vi "Conf Alarm.vi"(0 "VISA Resource Name":refnum<visa-resource-name>, 1 "Enable Alarm? (T:Enable)":bool=TRUE, 2 "Set/Check (F:Set)":bool, 3 "Polarity (T:Positive)":bool=TRUE, 4 "Mode (F:Track)":bool, 5 "error in (no error)":errorcluster, 6 "Alarm(s) (2:Both)":enum16{"Lower", "Upper", "Both"}(ring)=enum."Both", 7 "Lower Limit (0)":dbl format="%.2f", 8 "Channel List(empty)":string, 9 "Upper Limit (0)":dbl format="%.2f", 10 "Check (2:Lower Limit)":T1(ring)=enum."Lower Limit", 11 "Clear Bit (5:None)":enum16{"1", "2", "3", "4", "All", "None"}(ring)=enum."None", 13 "Output # (1)":enum16{"1", "2", "3", "4"}(ring)) -> (14 "VISA Resource Name Out":refnum<visa-resource-name>, 16 "Configuration?":string, 19 "error out":errorcluster)   [LabVIEW 2012, in "Agilent 34970.lvlib"]
doc: "This VI lets you configure or check alarms on the specified analog channels."
uses:
  <instrlib>/Agilent 34970/Agilent 34970.lvlib
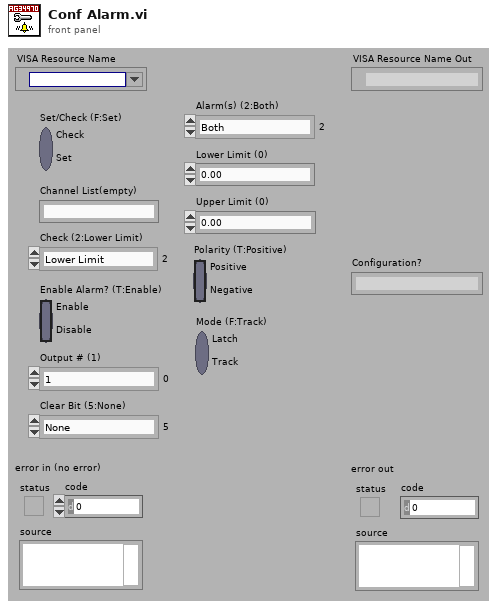
[diagram p1: front panel]
types:
  T1 = enum16{"Lower State", "Upper State", "Lower Limit", "Upper Limit", "Alarm #", "Polarity", "Mode"}
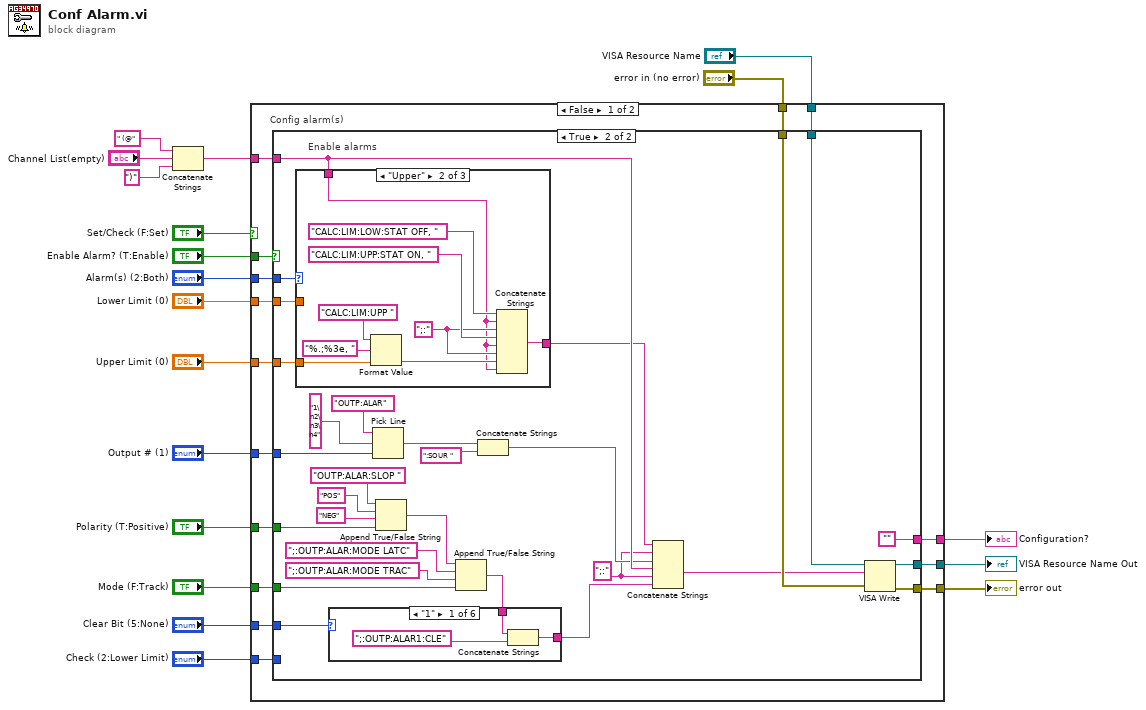
[diagram p0: block diagram]
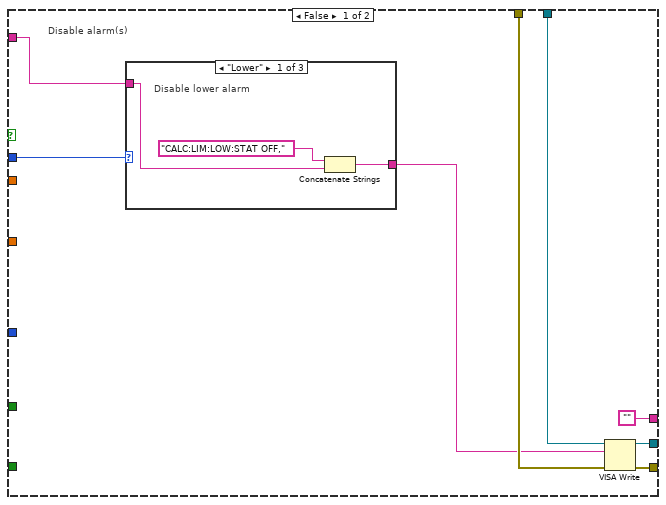
[diagram p2: hidden frame]
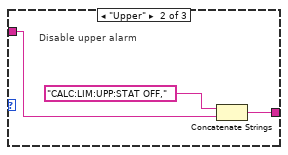
[diagram p3: hidden frame]
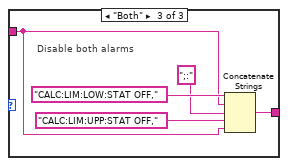
[diagram p4: hidden frame]
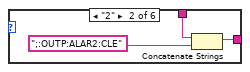
[diagram p5: hidden frame]
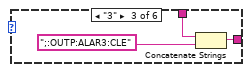
[diagram p6: hidden frame]
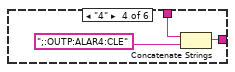
[diagram p7: hidden frame]
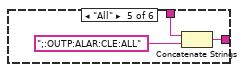
[diagram p8: hidden frame]
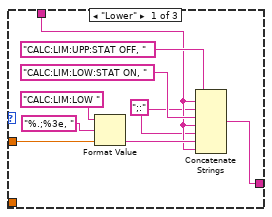
[diagram p10: hidden frame]
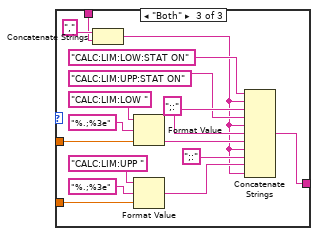
[diagram p11: hidden frame]
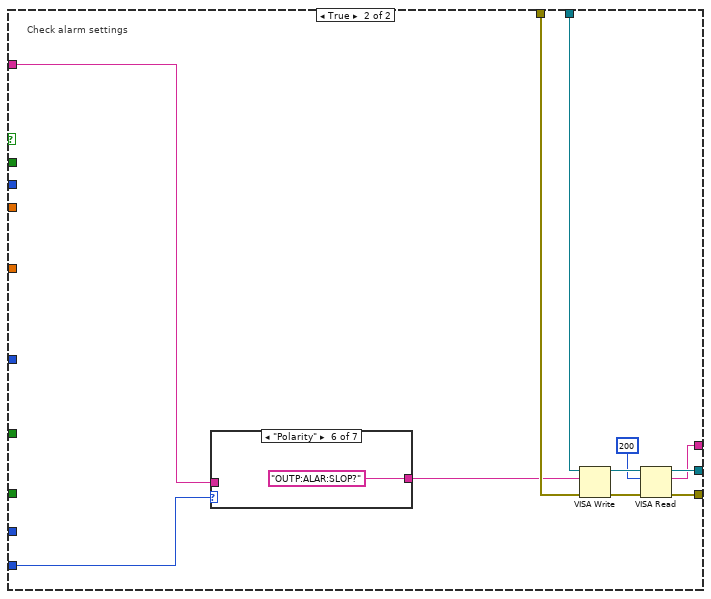
[diagram p12: hidden frame]
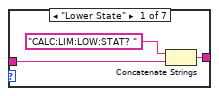
[diagram p13: hidden frame]
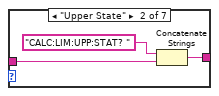
[diagram p14: hidden frame]
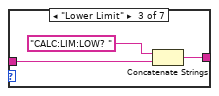
[diagram p15: hidden frame]
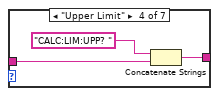
[diagram p16: hidden frame]
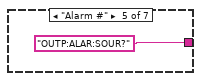
[diagram p17: hidden frame]
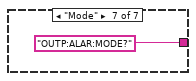
[diagram p18: hidden frame]
diagram:
  n1 = Concatenate Strings(" (@", "Channel List(empty)", ")") -> (w16:string)
  n2 = case shown="False" "Set/Check (F:Set)" {
    tunnel: w16 -> [w34 w135]
    tunnel: "error in (no error)" -> [w33 w140]
    tunnel: "VISA Resource Name" -> [w32 w139]
    tunnel: [w31 w138] -> w4
    tunnel: [w30 w136] -> w3
    tunnel: [w29 w137] -> w15
    tunnel: "Alarm(s) (2:Both)" -> [w28 _]
    tunnel: "Lower Limit (0)" -> [w27 _]
    tunnel: "Upper Limit (0)" -> [w26 _]
    tunnel: "Output # (1)" -> [w25 _]
    tunnel: "Polarity (T:Positive)" -> [w24 _]
    tunnel: "Mode (F:Track)" -> [w23 _]
    tunnel: "Clear Bit (5:None)" -> [w22 _]
    tunnel: "Check (2:Lower Limit)" -> [w21 w133]
    tunnel: "Enable Alarm? (T:Enable)" -> [w20 _]
    frame False {
      # "Config alarm(s)"
      n3 = case shown="True" w20 {
        tunnel: w34 -> [w37 w62]
        tunnel: w33 -> [w39 w82]
        tunnel: w32 -> [w38 w81]
        tunnel: [w41 w80] -> w31
        tunnel: [w40 w79] -> w30
        tunnel: ["" ""] -> w29
        tunnel: w28 -> [w36 w77]
        tunnel: w27 -> [_ w76]
        tunnel: w26 -> [_ w75]
        tunnel: w25 -> [_ w72]
        tunnel: w24 -> [_ w68]
        tunnel: w23 -> [_ w66]
        tunnel: w22 -> [_ w65]
        tunnel: w21 -> [_ _]
        frame False {
          # "Disable alarm(s)"
          n4 = case shown="\"Lower\"" w36 {
            tunnel: [w44 w47 w50] -> w35
            tunnel: w37 -> [w43 w46 w49]
            frame "Lower" {
              # "Disable lower alarm"
              n5 = Concatenate Strings("CALC:LIM:LOW:STAT OFF,", w43) -> (w44:string)
            }
            frame "Upper" {
              # "Disable upper alarm"
              n6 = Concatenate Strings("CALC:LIM:UPP:STAT OFF,", w46) -> (w47:string)
            }
            frame "Both" {
              # "Disable both alarms"
              n7 = Concatenate Strings("CALC:LIM:LOW:STAT OFF,", w49, ";:", "CALC:LIM:UPP:STAT OFF,", w49) -> (w50:string)
            }
          }
          n8 = VISA Write(VISA resource name=w38, write buffer=w35, error in (no error)=w39) -> (VISA resource name out=w41:refnum<visa-resource-name>, error out=w40:errorcluster)  [unwired: 1 out]
        }
        frame True {
          w60 = ";:"
          # "Enable alarms"
          n9 = case shown="\"Upper\"" w77 {
            tunnel: w76 -> [w106 _ w130]
            tunnel: w75 -> [_ w112 w129]
            tunnel: w62 -> [w101 w108 w119]
            tunnel: [w103 w111 w117] -> w59
            frame "Lower" {
              w100 = ";:"
              n10 = Format Value(string ("")="CALC:LIM:LOW ", format string="%.;%3e, ", value (0)=w106) -> (output string=w105:string)
              n11 = Concatenate Strings("CALC:LIM:UPP:STAT OFF, ", w101, w100, "CALC:LIM:LOW:STAT ON, ", w101, w100, w105, w101) -> (w103:string)
            }
            frame "Upper" {
              w109 = ";:"
              n12 = Format Value(string ("")="CALC:LIM:UPP ", format string="%.;%3e, ", value (0)=w112) -> (output string=w114:string)
              n13 = Concatenate Strings("CALC:LIM:LOW:STAT OFF, ", w108, w109, "CALC:LIM:UPP:STAT ON, ", w108, w109, w114, w108) -> (w111:string)
            }
            frame "Both" {
              w123 = ";:"
              n14 = Concatenate Strings(",", w119) -> (w118:string)
              n15 = Format Value(string ("")="CALC:LIM:LOW ", format string="%.;%3e", value (0)=w130) -> (output string=w126:string)
              n16 = Format Value(string ("")="CALC:LIM:UPP ", format string="%.;%3e", value (0)=w129) -> (output string=w124:string)
              n17 = Concatenate Strings("CALC:LIM:LOW:STAT ON", w118, w123, "CALC:LIM:UPP:STAT ON", w118, w123, w126, w118, ";:", w124, w118) -> (w117:string)
            }
          }
          n18 = Pick Line(string ("")="OUTP:ALAR", multi-line string="1\n2\n3\n4", line index=w72) -> (output string=w71:string)
          n19 = Append True/False String(1:w68, 2:"NEG", 3:"POS", 4:"OUTP:ALAR:SLOP ") -> (0:w67:string)
          n20 = Append True/False String(1:w66, 2:";:OUTP:ALAR:MODE TRAC", 3:";:OUTP:ALAR:MODE LATC", 4:w67) -> (0:w64:string)
          n21 = case shown="\"1\"" w65 {
            tunnel: w64 -> [w85 w87 w90 w93 w96 w98]
            tunnel: [w83 w86 w89 w92 w95 w98] -> w63
            frame "1" {
              n22 = Concatenate Strings(w85, ";:OUTP:ALAR1:CLE") -> (w83:string)
            }
            frame "2" {
              n23 = Concatenate Strings(w87, ";:OUTP:ALAR2:CLE") -> (w86:string)
            }
            frame "3" {
              n24 = Concatenate Strings(w90, ";:OUTP:ALAR3:CLE") -> (w89:string)
            }
            frame "4" {
              n25 = Concatenate Strings(w93, ";:OUTP:ALAR4:CLE") -> (w92:string)
            }
            frame "All" {
              n26 = Concatenate Strings(w96, ";:OUTP:ALAR:CLE:ALL") -> (w95:string)
            }
            frame "None" {
            }
          }
          n27 = Concatenate Strings(w71, ":SOUR ") -> (w61:string)
          n28 = Concatenate Strings(w59, w60, w61, w62, w60, w63) -> (w56:string)
          n29 = VISA Write(VISA resource name=w81, write buffer=w56, error in (no error)=w82) -> (VISA resource name out=w80:refnum<visa-resource-name>, error out=w79:errorcluster)  [unwired: 1 out]
        }
      }
    }
    frame True {
      # "Check alarm settings"
      n30 = case shown="\"Polarity\"" w133 {
        tunnel: [w145 w148 w151 w154 "OUTP:ALAR:SOUR?" "OUTP:ALAR:SLOP?" "OUTP:ALAR:MODE?"] -> w134
        tunnel: w135 -> [w144 w147 w150 w153 _ _ _]
        frame "Lower State" {
          n31 = Concatenate Strings("CALC:LIM:LOW:STAT? ", w144) -> (w145:string)
        }
        frame "Upper State" {
          n32 = Concatenate Strings("CALC:LIM:UPP:STAT? ", w147) -> (w148:string)
        }
        frame "Lower Limit" {
          n33 = Concatenate Strings("CALC:LIM:LOW? ", w150) -> (w151:string)
        }
        frame "Upper Limit" {
          n34 = Concatenate Strings("CALC:LIM:UPP? ", w153) -> (w154:string)
        }
        frame "Alarm #" {
        }
        frame "Polarity" {
        }
        frame "Mode" {
        }
      }
      n35 = VISA Write(VISA resource name=w139, write buffer=w134, error in (no error)=w140) -> (VISA resource name out=w142:refnum<visa-resource-name>, error out=w143:errorcluster)  [unwired: 1 out]
      n36 = VISA Read(VISA resource name=w142, byte count=u32 200 ("byte count (0)"), error in (no error)=w143) -> (VISA resource name out=w138:refnum<visa-resource-name>, read buffer=w137:string, error out=w136:errorcluster)  [unwired: 1 out]
    }
  }
  "Configuration?" <- w15
  "VISA Resource Name Out" <- w4
  "error out" <- w3
